vi "Get All Config.vi"(8 "error in (no error)":errorcluster, 10 "Main Ctr in":T1={"Tite"="", "Base path"=path "", "Table"=[], "Stations"=[], "Shield Array"=[], "UPHs"=[], "VISA"={"VISA"="", "baud rate"=9600, "data bits"=8, "parity"=enum."None", "stop bits"=10, "flow control"=0}, "Path"={"roof"=path "", "Config"=path "", "Png"=path ""}, "Ctr"={"DB Dispaly"=refnum, "Error Table"=refnum, "Display"=refnum, "Login"=refnum, "Exit"=refnum, "FTT_Submit"=refnum}, "Login"={"User"="", "Grade"=""}, "information"={"cause"="", "Type"=enum."Inform", "code"=0, "Suroce"="", "Status"=FALSE}, "Local DB"={"Connstr"="", "Database"={"Constr"={"Driver"="", "Server"="", "User"="", "Pwd"="", "Database"=""}, "conn ref"=refnum, "State"=FALSE}}, "Remote DB"={"Connstr"="", "Database"={"Constr"={"Driver"="", "Server"="", "User"="", "Pwd"="", "Database"=""}, "conn ref"=refnum, "State"=FALSE}}, "FTT TV"="", "ExchangeTime"=0, "NVH"="", "EOL Path"=path ""} {"VISA"."flow control" items=["None", "XON/XOFF", "RTS/CTS", "XON/XOFF & RTS/CTS", "DTR/DSR", "XON/XOFF & DTR/DSR"]; "VISA"."stop bits" items=["1.0"=10, "1.5"=15, "2.0"=20]}, 11 "Base Path":path=path "D:/Inalfa_Work/Project Program/FTT_Project/TP3_FTT") -> (0 "error out":errorcluster, 3 "Cluster":T1={"Tite"="", "Base path"=path "", "Table"=[], "Stations"=[], "Shield Array"=[], "UPHs"=[], "VISA"={"VISA"="", "baud rate"=9600, "data bits"=8, "parity"=enum."None", "stop bits"=10, "flow control"=0}, "Path"={"roof"=path "", "Config"=path "", "Png"=path ""}, "Ctr"={"DB Dispaly"=refnum, "Error Table"=refnum, "Display"=refnum, "Login"=refnum, "Exit"=refnum, "FTT_Submit"=refnum}, "Login"={"User"="", "Grade"=""}, "information"={"cause"="", "Type"=enum."Inform", "code"=0, "Suroce"="", "Status"=FALSE}, "Local DB"={"Connstr"="", "Database"={"Constr"={"Driver"="", "Server"="", "User"="", "Pwd"="", "Database"=""}, "conn ref"=refnum, "State"=FALSE}}, "Remote DB"={"Connstr"="", "Database"={"Constr"={"Driver"="", "Server"="", "User"="", "Pwd"="", "Database"=""}, "conn ref"=refnum, "State"=FALSE}}, "FTT TV"="", "ExchangeTime"=0, "NVH"="", "EOL Path"=path ""} {"VISA"."flow control" items=["None", "XON/XOFF", "RTS/CTS", "XON/XOFF & RTS/CTS", "DTR/DSR", "XON/XOFF & DTR/DSR"]; "VISA"."stop bits" items=["1.0"=10, "1.5"=15, "2.0"=20]})   [LabVIEW 2014]
uses:
  Operation File/ini/type defs/ini file actions.ctl
  Operation File/ini/type defs/ini entry value.ctl
  Operation File/ini/type defs/ini entry types.ctl
  Operation File/ini/type defs/ini entry.ctl
  Type'def/UPH Config.ctl
  VISA/Ctr/VISA Ctr.ctl
  Type'def/MainCtr.ctl
  Type'def/Main Ctr Ref.ctl
  Type'def/User Login.ctl
  Database/Ctr/Constr.ctl
  <vilib>/addons/database/Connection.llb/Conn ObjectReference.ctl
  <vilib>/addons/database/NI_Database_API.lvlib
  Database/Ctr/Conneect State.ctl
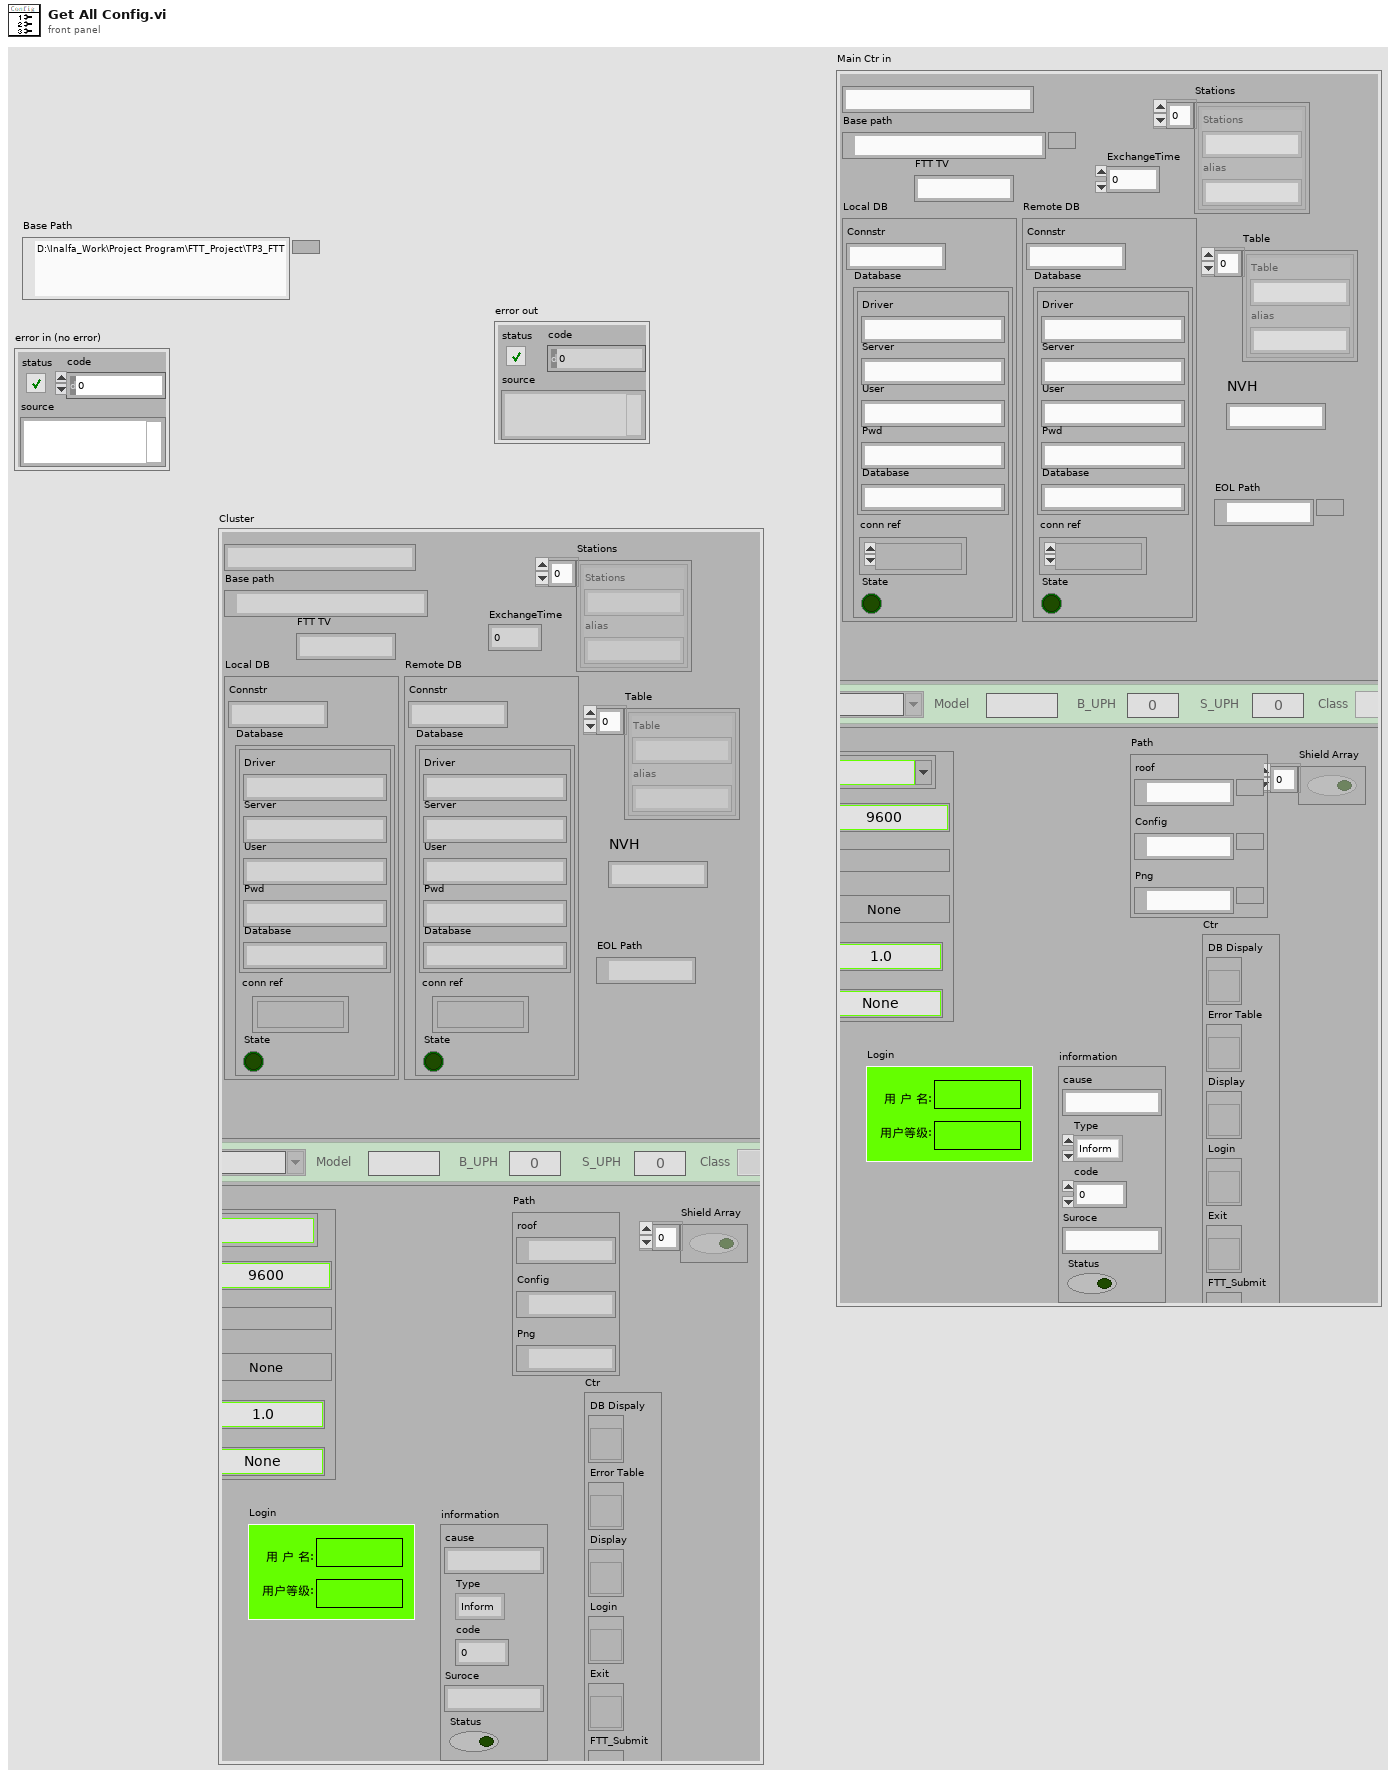
[diagram p1: front panel]
types:
  T1 = typedef "MainCtr.ctl" = cluster{"Tite":string, "Base path":path, "Table":cluster{"Table":string, "alias":string}[], "Stations":cluster{"Stations":string, "alias":string}[], "Shield Array":bool[], "UPHs":T2[], "VISA":T3, "Path":cluster{"roof":path, "Config":path, "Png":path}, "Ctr":T4, "Login":T5, "information":cluster{"cause":string, "Type":enum16{"Inform", "Warning", "Alarm"}, "code":i32, "Suroce":string, "Status":bool}, "Local DB":cluster{"Connstr":string, "Database":T6}, "Remote DB":cluster{"Connstr":string, "Database":T6}, "FTT TV":string, "ExchangeTime":i32, "NVH":string, "EOL Path":path}
  T2 = typedef "UPH Config.ctl" = cluster{"Line_No":string, "Model":string, "B_UPH ":i16, "S_UPH  ":i16, "Class":enum16{"Big", "Small"}}
  T3 = typedef "VISA Ctr.ctl" = cluster{"VISA":refnum<visa-resource-name>, "baud rate":u32, "data bits":u16, "parity":enum16{"None", "Odd", "Even", "Mark", "Space"}, "stop bits":u16, "flow control":u16}
  T4 = typedef "Main Ctr Ref.ctl" = cluster{"DB Dispaly":refnum<vi>, "Error Table":refnum<vi>, "Display":refnum<vi>, "Login":refnum<vi>, "Exit":refnum<vi>, "FTT_Submit":refnum<vi>}
  T5 = typedef "User Login.ctl" = cluster{"User":string, "Grade":string}
  T6 = typedef "Conneect State.ctl" = cluster{"Constr":T7, "conn ref":T8, "State":bool}
  T7 = typedef "Constr.ctl" = cluster{"Driver":string, "Server":string, "User":string, "Pwd":string, "Database":string}
  T8 = typedef "NI_Database_API.lvlib/Conn ObjectReference.ctl" = refnum<k1>
  T9 = typedef "ini entry.ctl" = cluster{"section":string, "key":string, "type":T10, "default value":T11}
  T10 = typedef "ini entry types.ctl" = enum16{"Boolean", "Double", "I32", "Path", "String", "U32"}
  T11 = typedef "ini entry value.ctl" = cluster{"Boolean":bool, "Dbl":dbl, "I32":i32, "Path":path, "String":string, "U32":u32}
  T12 = typedef "ini file actions.ctl" = enum16{"read ini", "write ini"}
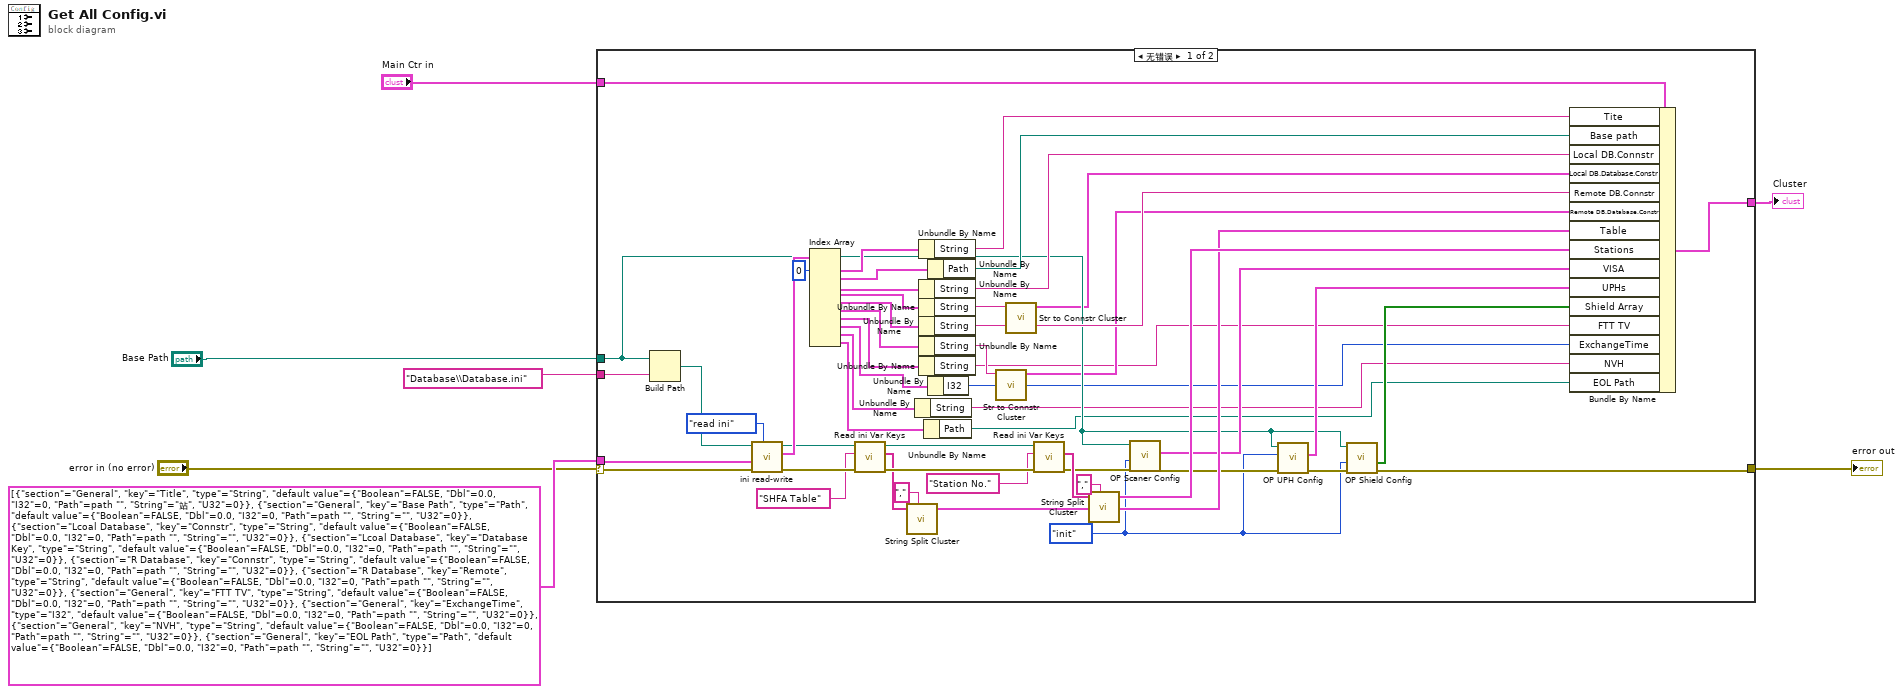
[diagram p0: block diagram]
diagram:
  n1 = case shown="无错误" "error in (no error)" {
    selector: "error in (no error)" -> [w59 w60]
    tunnel: [w22 w60] -> w7
    tunnel: T9[] [{"section"="General", "key"="Title", "type"=enum."String", "default value"={"Boolean"=FALSE, "Dbl"=0.0, "I32"=0, "Path"=path "", "String"="站", "U32"=0}}, {"section"="General", "key"="Base Path", "type"=enum."Path", "default value"={"Boolean"=FALSE, "Dbl"=0.0, "I32"=0, "Path"=path "", "String"="", "U32"=0}}, {"section"="Lcoal Database", "key"="Connstr", "type"=enum."String", "default value"={"Boolean"=FALSE, "Dbl"=0.0, "I32"=0, "Path"=path "", "String"="", "U32"=0}}, {"section"="Lcoal Database", "key"="Database Key", "type"=enum."String", "default value"={"Boolean"=FALSE, "Dbl"=0.0, "I32"=0, "Path"=path "", "String"="", "U32"=0}}, {"section"="R Database", "key"="Connstr", "type"=enum."String", "default value"={"Boolean"=FALSE, "Dbl"=0.0, "I32"=0, "Path"=path "", "String"="", "U32"=0}}, {"section"="R Database", "key"="Remote", "type"=enum."String", "default value"={"Boolean"=FALSE, "Dbl"=0.0, "I32"=0, "Path"=path "", "String"="", "U32"=0}}, {"section"="General", "key"="FTT TV", "type"=enum."String", "default value"={"Boolean"=FALSE, "Dbl"=0.0, "I32"=0, "Path"=path "", "String"="", "U32"=0}}, {"section"="General", "key"="ExchangeTime", "type"=enum."I32", "default value"={"Boolean"=FALSE, "Dbl"=0.0, "I32"=0, "Path"=path "", "String"="", "U32"=0}}, {"section"="General", "key"="NVH", "type"=enum."String", "default value"={"Boolean"=FALSE, "Dbl"=0.0, "I32"=0, "Path"=path "", "String"="", "U32"=0}}, {"section"="General", "key"="EOL Path", "type"=enum."Path", "default value"={"Boolean"=FALSE, "Dbl"=0.0, "I32"=0, "Path"=path "", "String"="", "U32"=0}}] ("ini entry descriptors") -> [w57 _]
    tunnel: "Main Ctr in" -> [w55 _]
    tunnel: [w34 _] -> w4
    tunnel: "Base Path" -> [w26 _]
    tunnel: "Database\\Database.ini" -> [w33 _]
    frame No Error {
      w25 = enum16{"init", "Read", "Write"}."init" ("Enum")
      n2 = Build Path(base path=w26, name or relative path=w33) -> (appended path=w32:path)
      n3 = call "ini read-write.vi"("action"=ini_file_actions."read ini", "error in (no error)"=w59, "ini entry descriptors"=w57, "configuration file path"=w32) -> ("error out"=w44:errorcluster, "values out"=w56:T11[], "configuration file path out"=w21:path)  [unwired: 5 in]
      n4 = Index Array(array=w56, index #1=0 ("索引")) -> (element #1=w54:T11, element #2=w52:T11, element #3=w50:T11, element #4=w48:T11, element #5=w47:T11, element #6=w45:T11, element #7=w16:T11, element #8=w13:T11, element #9=w11:T11, element #10=w9:T11)  [unwired: 9 in]
      n5 = call "Read ini Var Keys.vi"("error in (no error)"=w44, "section"="SHFA Table", "Base Path"=w21) -> ("error out"=w41:errorcluster, "Array"=w23:string[], "file path"=w40:path)  [unwired: 6 in]
      n6 = call "String Split Cluster.vi"("Array Str"=w23, "Char"=",") -> ("Array Cluster"=w35:cluster{"Table":string, "alias":string}[])  [unwired: 5 in]
      n7 = Unbundle By Name(w11) -> ("String"=w10:string)
      n8 = Unbundle By Name(w54) -> ("String"=w53:string)
      n9 = Unbundle By Name(w50) -> ("String"=w49:string)
      n10 = Unbundle By Name(w48) -> ("String"=w20:string)
      n11 = Unbundle By Name(w47) -> ("String"=w46:string)
      n12 = Unbundle By Name(w45) -> ("String"=w18:string)
      n13 = Unbundle By Name(w16) -> ("String"=w15:string)
      n14 = Unbundle By Name(w9) -> ("Path"=w8:path)
      n15 = Unbundle By Name(w52) -> ("Path"=w51:path)
      n16 = Unbundle By Name(w13) -> ("I32"=w12:i32)
      n17 = call "Str to Connstr Cluster.vi"("Connstr"=w18) -> ("output cluster"=w17:T7)  [unwired: 10 in]
      n18 = call "Str to Connstr Cluster.vi"("Connstr"=w20) -> ("output cluster"=w19:T7)  [unwired: 10 in]
      n19 = call "Read ini Var Keys.vi"("error in (no error)"=w41, "section"="Station No.", "Base Path"=w40) -> ("error out"=w31:errorcluster, "Array"=w37:string[])  [unwired: 6 in, 1 out]
      n20 = call "String Split Cluster.vi"("Array Str"=w37, "Char"=",") -> ("Array Cluster"=w36:cluster{"Table":string, "alias":string}[])  [unwired: 5 in]
      n21 = call "OP Scaner Config.vi"("error in (no error)"=w31, "Enum"=w25, "Path"=w26) -> ("error out"=w29:errorcluster, "VISA"=w30:T3)  [unwired: 6 in, 1 out]
      n22 = call "OP UPH Config.vi"("error in (no error)"=w29, "Enum"=w25, "Path"=w26) -> ("error out"=w27:errorcluster, "UPH out"=w28:T2[])  [unwired: 6 in, 1 out]
      n23 = call "OP Shield Config.vi"("error in (no error)"=w27, "Enum"=w25, "Path"=w26) -> ("error out"=w22:errorcluster, "subarray"=w24:bool[])  [unwired: 5 in, 2 out]
      n24 = Bundle By Name(cluster=w55, "Tite"=w53, "Base path"=w51, "Local DB.Connstr"=w49, "Local DB.Database.Constr"=w19, "Remote DB.Connstr"=w46, "Remote DB.Database.Constr"=w17, "Table"=w35, "Stations"=w36, "VISA"=w30, "UPHs"=w28, "Shield Array"=w24, "FTT TV"=w15, "ExchangeTime"=w12, "NVH"=w10, "EOL Path"=w8) -> (w34:T1)
    }
    frame Error {
    }
  }
  "error out" <- w7
  "Cluster" <- w4
